vi "Write EEPROM data file.vi"(8 "error in (no error)":errorcluster, 9 "EEPROM files to write":string[](array[string]), 10 "client ptr":u32, 11 "Estyx device name":string) -> (0 "error out":errorcluster, 2 "To be written to the data file":string)   [LabVIEW 2010, in "lib1299.lvlib"]
doc: "This VI reads the contents of the EEPROM located on the device EVM (daughtercard).\n\nInputs:\nclient ptr - estyx client pointer to file system\nestyx device name - estyx directory name of the device\nTest mode (debug) - allow for testing without EEPROM input. User must supply string to parse.\n\nOutputs:\nRead Data - cluster of information read from the EEPROM\n - Raw Data: contents of eepage 1 date file from estyx\n - Parsed Data: Raw Data parsed based on memory range for the data value (defined on wiki page for EEPROM information)\n - Data - String: EEPROM data derived from finding the string terminator for each of the Parse Data lines"
uses:
  lib1299.lvlib
  Styx/lvstyx/Write/lvstyx_write_path_int.vi
  Styx/lvstyx/Write/lvstyx_write_path.vi
panel:
  out "ASCII Array":i32[][](array[numeric]) format="%.0x"
  # "Device Name"
  # "PWB EDGE number and rev"
  # "PCA EDGE number and rev"
  # "BOM EDGE number and rev"
  # "Build Date"
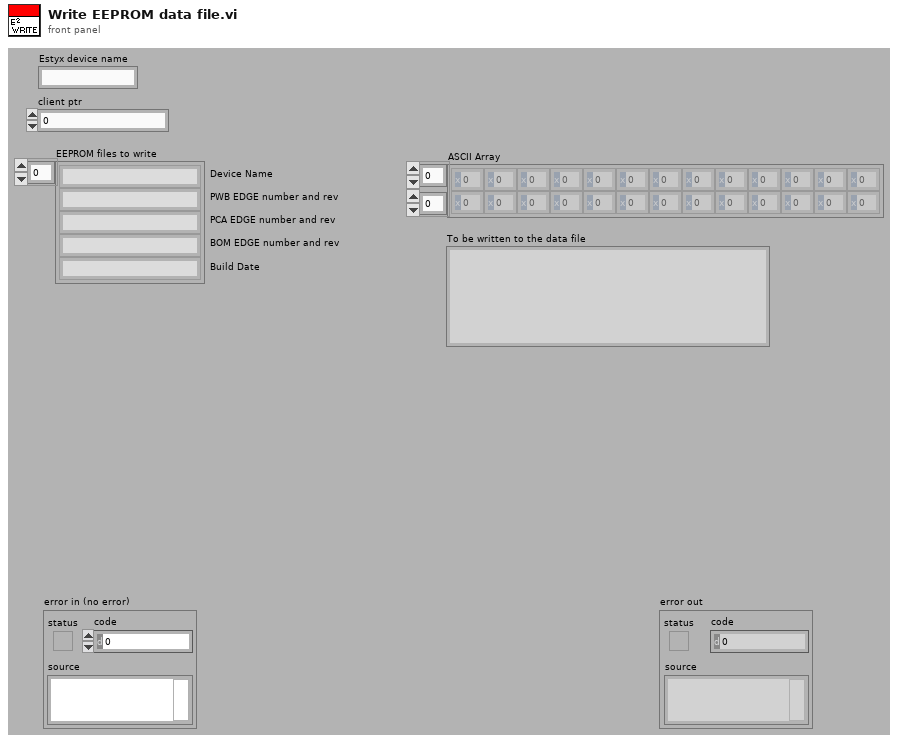
[diagram p1: front panel]
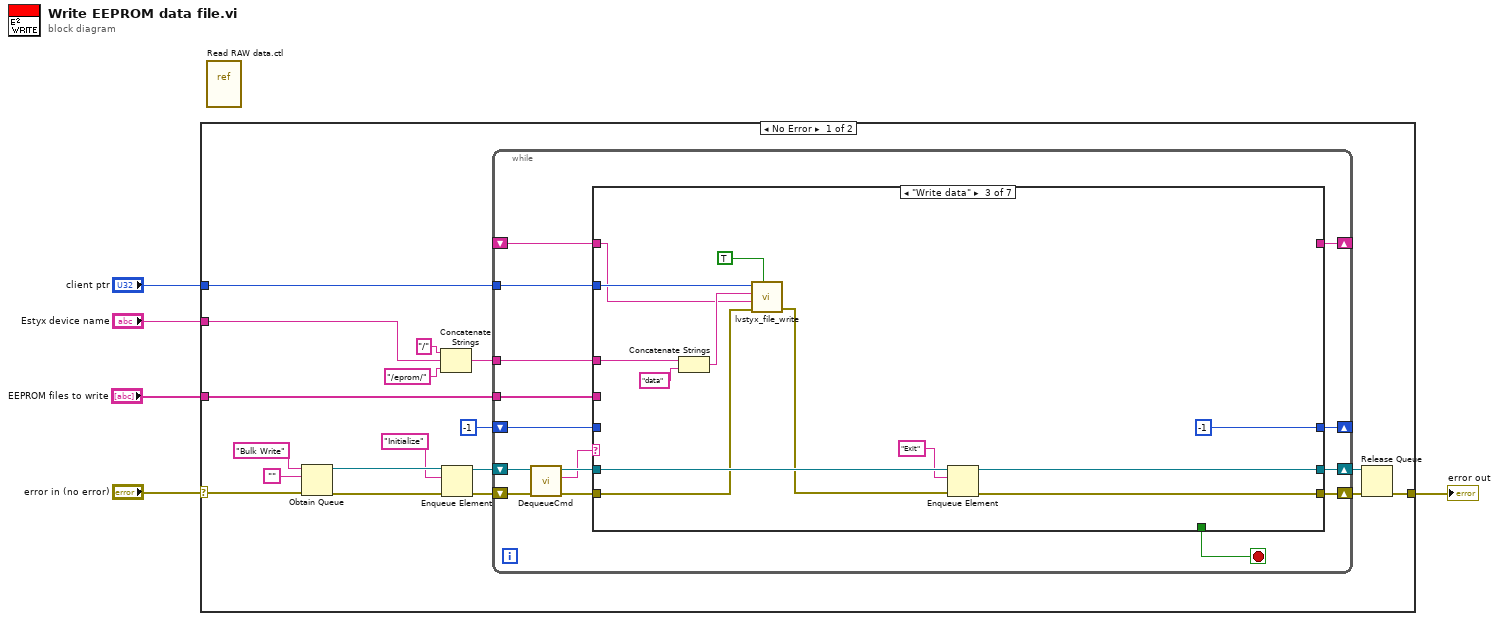
[diagram p0: block diagram]
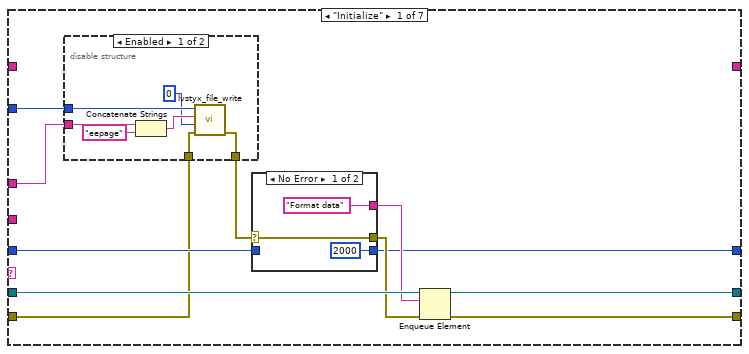
[diagram p2: hidden frame]
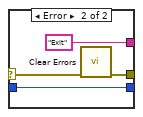
[diagram p4: hidden frame]
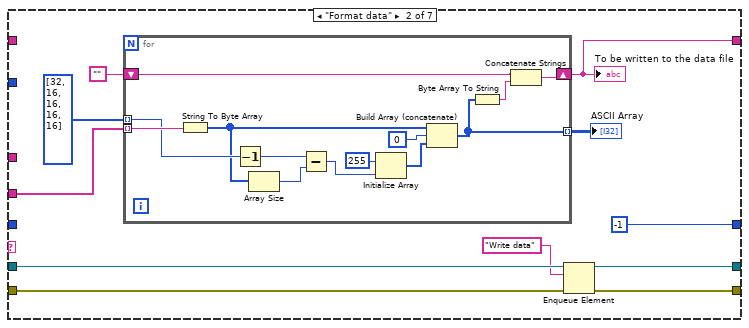
[diagram p5: hidden frame]
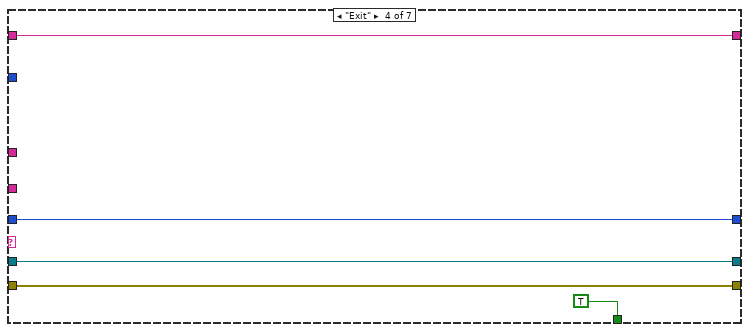
[diagram p6: hidden frame]
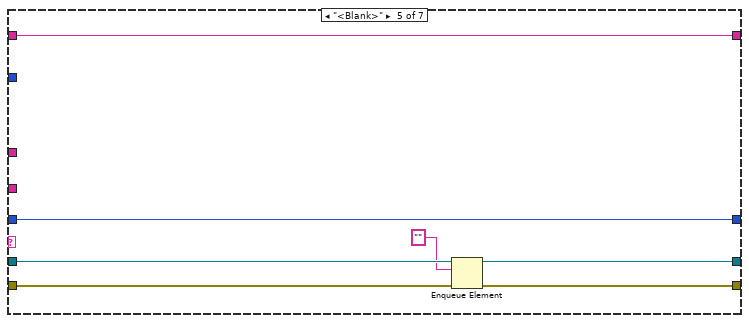
[diagram p7: hidden frame]
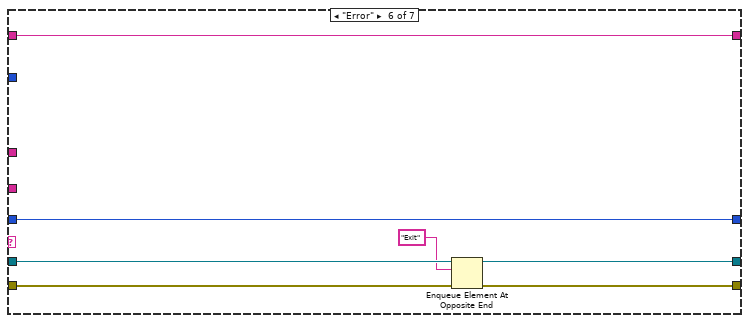
[diagram p8: hidden frame]
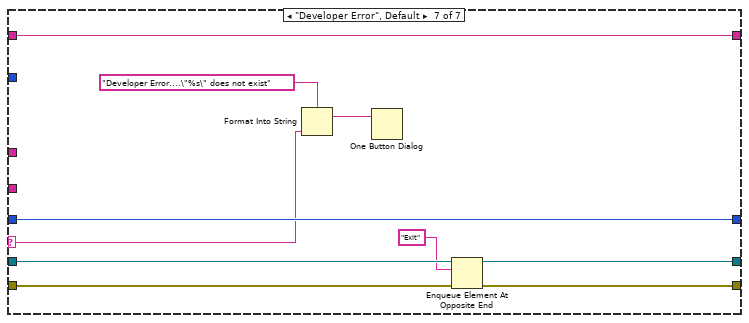
[diagram p9: hidden frame]
diagram:
  n1 = case shown="No Error" "error in (no error)" {
    selector: "error in (no error)" -> [w8 w131]
    tunnel: "Estyx device name" -> [w21 _]
    tunnel: "client ptr" -> [w14 _]
    tunnel: [w9 w131] -> w3
    tunnel: "EEPROM files to write" -> [w6 _]
    frame No Error {
      n2 = Obtain Queue(name (unnamed)="Bulk Write", element data type="", error in (no error)=w8) -> (queue out=w18:refnum<queue>, error out=w17:errorcluster)  [unwired: 2 in, 1 out]
      n3 = Concatenate Strings("/" ("string"), w21, "/eprom/" ("string")) -> (w13:string)
      n4 = Enqueue Element(queue=w18, element="Initialize", error in (no error)=w17) -> (queue out=w16:refnum<queue>, error out=w15:errorcluster)  [unwired: 1 in, 1 out]
      n5 = while {
        shift-right: [w34] -> w11
        shift-left: w15 -> [w37]
        shift-right: [w28] -> w10
        shift-left: w16 -> [w38]
        tunnel: w14 -> [w32]
        tunnel: w13 -> [w31]
        shift-right: [w29] -> _
        shift-left: -1 -> [w30]
        shift-right: [w27] -> _
        shift-left: _ -> [w26]
        tunnel: w6 -> [w24]
        stop <- w25 stop-if-true
        n6 = call <userlib>:"DequeueCmd.vi"("error in (no error)"=w37, "queue of text strings"=w38) -> ("error out"=w35:errorcluster, "command"=w33:string, "queue (dup)"=w36:refnum<queue>)  [unwired: 6 in, 1 out]
        n7 = case shown="\"Write data\"" w33 {
          selector: w33 -> [_ _ _ _ _ _ w122]
          tunnel: w36 -> [w48 w73 w97 w105 w111 w118 w128]
          tunnel: w35 -> [w40 w68 w93 w104 w113 w120 w130]
          tunnel: [w45 w75 w99 w104 w112 w119 w129] -> w34
          tunnel: w32 -> [w41 _ w94 _ _ _ _]
          tunnel: w31 -> [w49 _ w100 _ _ _ _]
          tunnel: w30 -> [w44 _ _ w106 w108 w115 w125]
          tunnel: [w43 -1 -1 w106 w108 w115 w125] -> w29
          tunnel: [w42 w74 w98 w105 w109 w116 w126] -> w28
          tunnel: [_ w65 _ w102 w107 w114 w124] -> w27
          tunnel: w26 -> [_ _ w90 w102 w107 w114 w124]
          tunnel: [_ _ _ TRUE _ _ _] -> w25
          tunnel: w24 -> [_ w70 _ _ _ _ _]
          frame "Initialize" {
            n8 = disable-structure shown="Enabled" {
              disable-tunnel: w49 -> [w56 _]
              disable-tunnel: w41 -> [w54 _]
              disable-tunnel: w40 -> [w51 w57]
              disable-tunnel: [w50 w57] -> w39
              frame Enabled {
                n9 = Concatenate Strings(w56, "eepage" ("string")) -> (w53:string)
                n10 = call-poly "lvstyx_file_write.vi"("error in (no error)"=w51, "int64"=i64 0, "path"=w53, "client ptr"=w54) -> ("error out"=w50:errorcluster)  [unwired: 6 in, 1 out]
              }
              frame Disabled {
              }
            }
            n11 = case shown="No Error" w39 {
              selector: w39 -> [w59 w63]
              tunnel: ["Format data" ("element") "Exit" ("element")] -> w46
              tunnel: [w59 w62] -> w47
              tunnel: w44 -> [_ w61]
              tunnel: [2000 w61] -> w43
              frame No Error {
              }
              frame Error {
                n12 = call <vilib>:"Clear Errors.vi"("error in (no error)"=w63) -> ("error out"=w62:errorcluster)  [unwired: 6 in]
              }
            }
            n13 = Enqueue Element(queue=w48, element=w46, error in (no error)=w47) -> (queue out=w42:refnum<queue>, error out=w45:errorcluster)  [unwired: 1 in, 1 out]
          }
          frame "Format data" {
            n14 = for {
              tunnel: w70 -> [w88] mode=indexing
              tunnel: i32[] [32, 16, 16, 16, 16] -> [w87] mode=indexing
              tunnel: [w83] -> w67 mode=indexing
              shift-right: [w81] -> w65
              shift-left: "" -> [w82]
              n15 = String To Byte Array(string=w88) -> (unsigned byte array=w84:u8[])
              n16 = Decrement(x=w87) -> (x-1=w85:i32)
              n17 = Array Size(array=w84) -> (size(s)=w86:i32)
              n18 = Subtract(x=w85, y=w86) -> (x-y=w77:i32)
              n19 = Initialize Array(u8 255 ("dimension size"), w77) -> (w79:u8[])
              n20 = Build Array (concatenate)(w84, u8 0, w79) -> (w83:u8[])
              n21 = Byte Array To String(unsigned byte array=w83) -> (string=w80:string)
              n22 = Concatenate Strings(w82, w80) -> (w81:string)
            }
            "To be written to the data file" <- w65
            "ASCII Array" <- w67
            n23 = Enqueue Element(queue=w73, element="Write data", error in (no error)=w68) -> (queue out=w74:refnum<queue>, error out=w75:errorcluster)  [unwired: 1 in, 1 out]
          }
          frame "Write data" {
            n24 = Concatenate Strings(w100, "data" ("string")) -> (w91:string)
            n25 = call-poly "lvstyx_file_write.vi"("Log? (T)"=TRUE ("Notify? (F)"), "error in (no error)"=w93, "buf"=w90, "path"=w91, "client ptr"=w94) -> ("error out"=w92:errorcluster)  [unwired: 4 in, 2 out]
            n26 = Enqueue Element(queue=w97, element="Exit", error in (no error)=w92) -> (queue out=w98:refnum<queue>, error out=w99:errorcluster)  [unwired: 1 in, 1 out]
          }
          frame "Exit" {
          }
          frame "<Blank>" {
            n27 = Enqueue Element(queue=w111, element="", error in (no error)=w113) -> (queue out=w109:refnum<queue>, error out=w112:errorcluster)  [unwired: 1 in, 1 out]
          }
          frame "Error" {
            n28 = Enqueue Element At Opposite End(queue=w118, element="Exit", error in (no error)=w120) -> (queue out=w116:refnum<queue>, error out=w119:errorcluster)  [unwired: 1 in, 1 out]
          }
          frame "Developer Error", Default {
            n29 = Format Into String(format string="Developer Error....\"%s\" does not exist", w122) -> (resulting string=w123:string)  [unwired: 2 in, 1 out]
            n30 = One Button Dialog(message=w123) -> ()  [unwired: 1 in, 1 out]
            n31 = Enqueue Element At Opposite End(queue=w128, element="Exit", error in (no error)=w130) -> (queue out=w126:refnum<queue>, error out=w129:errorcluster)  [unwired: 1 in, 1 out]
          }
        }
      }
      n32 = Release Queue(queue=w10, error in (no error)=w11) -> (error out=w9:errorcluster)  [unwired: 1 in, 2 out]
    }
    frame Error {
    }
  }
  "error out" <- w3
  n33 = vi-ref "Read RAW data.ctl"() -> ()  [unwired: 1 out]
